vi "MGCC_FntStaMach_Control panel loop.vi"   [LabVIEW 2016]
doc: "This VI is used to convert the flags into events."
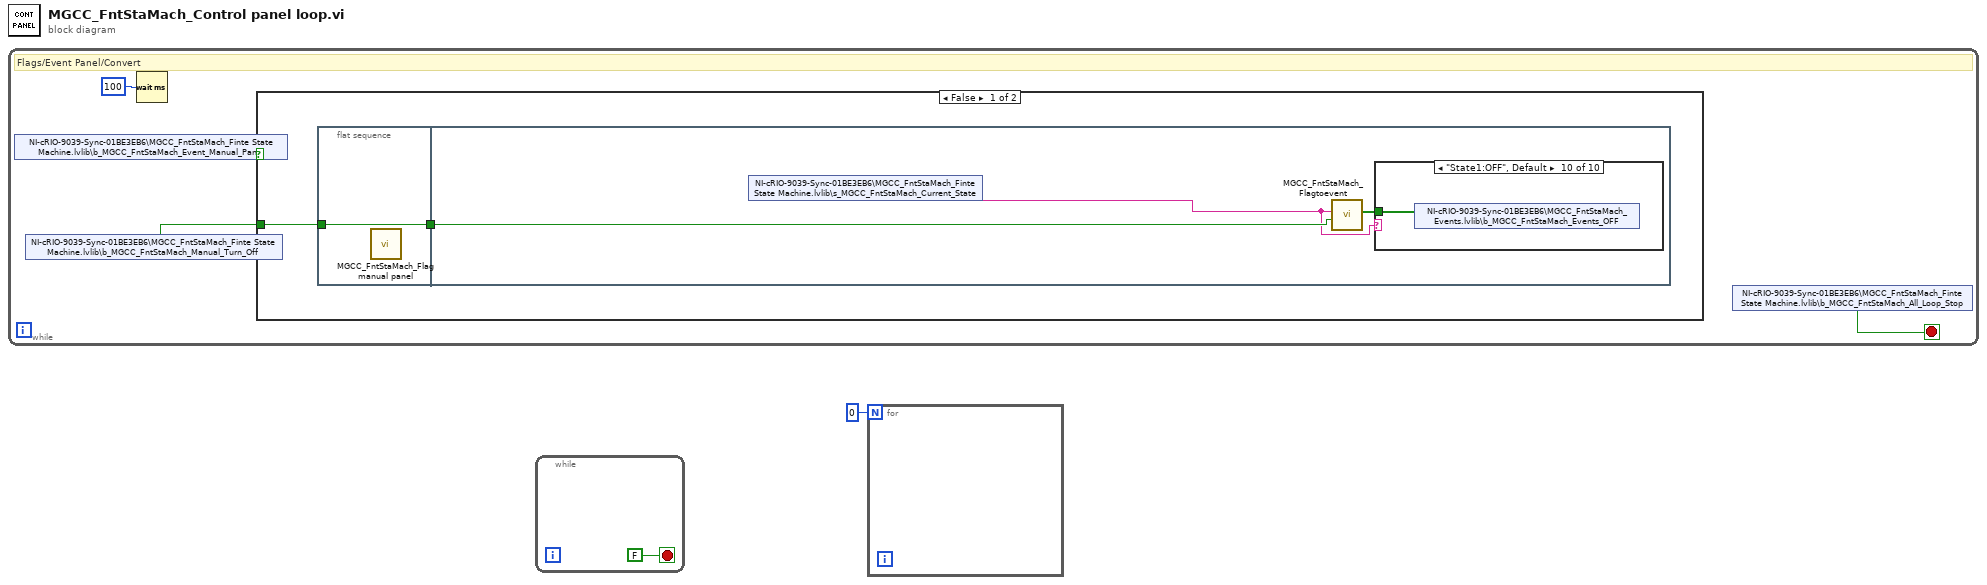
[diagram p0: block diagram]
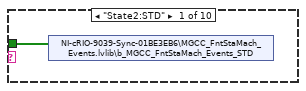
[diagram p2: hidden frame]
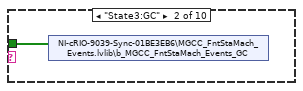
[diagram p3: hidden frame]
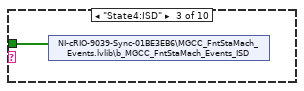
[diagram p4: hidden frame]
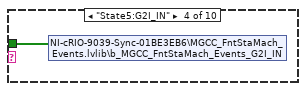
[diagram p5: hidden frame]
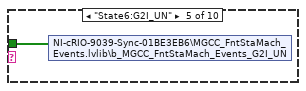
[diagram p6: hidden frame]
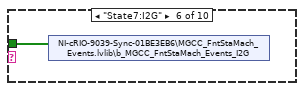
[diagram p7: hidden frame]
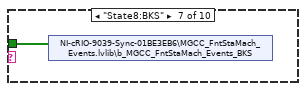
[diagram p8: hidden frame]
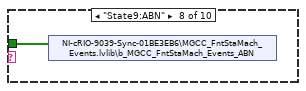
[diagram p9: hidden frame]
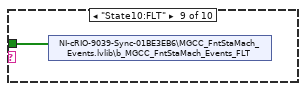
[diagram p10: hidden frame]
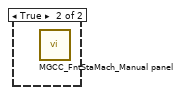
[diagram p11: hidden frame]
diagram:
  n1 = while {
    stop <- w4 stop-if-true
    # "Flags/Event Panel/Convert"
    n2 = shared-variable "NI-cRIO-9039-Sync-01BE3EB6\\MGCC_FntStaMach_Finte State Machine.lvlib\\b_MGCC_FntStaMach_Event_Manual_Panel"() -> (w3:bool)  [unwired: 1 in, 1 out]
    n3 = shared-variable "NI-cRIO-9039-Sync-01BE3EB6\\MGCC_FntStaMach_Finte State Machine.lvlib\\b_MGCC_FntStaMach_Manual_Turn_Off"() -> (w2:bool)  [unwired: 1 in, 1 out]
    n4 = Wait (ms)(milliseconds to wait=u32 100) -> ()  [unwired: 1 out]
    n5 = case shown="False" w3 {
      tunnel: w2 -> [w7 _]
      frame False {
        n6 = flat-sequence {
          tunnel: w7 -> [w8]
          tunnel: [w8] -> w6
          tunnel: w6 -> [w11]
          frame #0 {
            n7 = call "MGCC_FntStaMach_Flag manual panel.vi"() -> ()  [unwired: 12 in]
          }
          frame #1 {
            n8 = shared-variable "NI-cRIO-9039-Sync-01BE3EB6\\MGCC_FntStaMach_Finte State Machine.lvlib\\s_MGCC_FntStaMach_Current_State"() -> (w9:string)  [unwired: 1 in, 1 out]
            n9 = call "MGCC_FntStaMach_Flagtoevent.vi"("M_OFF"=w11, "Pre_state"=w9) -> ("Event"=w10:bool[])  [unwired: 9 in]
            n10 = case shown="\"State1:OFF\", Default" w9 {
              tunnel: w10 -> [w12 w13 w14 w15 w16 w17 w18 w19 w20 w21]
              frame "State2:STD" {
                n11 = shared-variable "NI-cRIO-9039-Sync-01BE3EB6\\MGCC_FntStaMach_Events.lvlib\\b_MGCC_FntStaMach_Events_STD"(w12) -> ()  [unwired: 1 in, 1 out]
              }
              frame "State3:GC" {
                n12 = shared-variable "NI-cRIO-9039-Sync-01BE3EB6\\MGCC_FntStaMach_Events.lvlib\\b_MGCC_FntStaMach_Events_GC"(w13) -> ()  [unwired: 1 in, 1 out]
              }
              frame "State4:ISD" {
                n13 = shared-variable "NI-cRIO-9039-Sync-01BE3EB6\\MGCC_FntStaMach_Events.lvlib\\b_MGCC_FntStaMach_Events_ISD"(w14) -> ()  [unwired: 1 in, 1 out]
              }
              frame "State5:G2I_IN" {
                n14 = shared-variable "NI-cRIO-9039-Sync-01BE3EB6\\MGCC_FntStaMach_Events.lvlib\\b_MGCC_FntStaMach_Events_G2I_IN"(w15) -> ()  [unwired: 1 in, 1 out]
              }
              frame "State6:G2I_UN" {
                n15 = shared-variable "NI-cRIO-9039-Sync-01BE3EB6\\MGCC_FntStaMach_Events.lvlib\\b_MGCC_FntStaMach_Events_G2I_UN"(w16) -> ()  [unwired: 1 in, 1 out]
              }
              frame "State7:I2G" {
                n16 = shared-variable "NI-cRIO-9039-Sync-01BE3EB6\\MGCC_FntStaMach_Events.lvlib\\b_MGCC_FntStaMach_Events_I2G"(w17) -> ()  [unwired: 1 in, 1 out]
              }
              frame "State8:BKS" {
                n17 = shared-variable "NI-cRIO-9039-Sync-01BE3EB6\\MGCC_FntStaMach_Events.lvlib\\b_MGCC_FntStaMach_Events_BKS"(w18) -> ()  [unwired: 1 in, 1 out]
              }
              frame "State9:ABN" {
                n18 = shared-variable "NI-cRIO-9039-Sync-01BE3EB6\\MGCC_FntStaMach_Events.lvlib\\b_MGCC_FntStaMach_Events_ABN"(w19) -> ()  [unwired: 1 in, 1 out]
              }
              frame "State10:FLT" {
                n19 = shared-variable "NI-cRIO-9039-Sync-01BE3EB6\\MGCC_FntStaMach_Events.lvlib\\b_MGCC_FntStaMach_Events_FLT"(w20) -> ()  [unwired: 1 in, 1 out]
              }
              frame "State1:OFF", Default {
                n20 = shared-variable "NI-cRIO-9039-Sync-01BE3EB6\\MGCC_FntStaMach_Events.lvlib\\b_MGCC_FntStaMach_Events_OFF"(w21) -> ()  [unwired: 1 in, 1 out]
              }
            }
          }
        }
      }
      frame True {
        n21 = call "MGCC_FntStaMach_Manual panel.vi"() -> ()  [unwired: 12 in]
      }
    }
    n22 = shared-variable "NI-cRIO-9039-Sync-01BE3EB6\\MGCC_FntStaMach_Finte State Machine.lvlib\\b_MGCC_FntStaMach_All_Loop_Stop"() -> (w4:bool)  [unwired: 1 in, 1 out]
  }
  n23 = while {
    stop <- FALSE stop-if-true
  }
  n24 = for {
    N: 0 -> [_]
  }
